vi "joystick+serial to robot.vi"() -> ()   [LabVIEW 2016]
uses:
  grSim/grSim Robot Command.ctl
  <vilib>/Instr/_visa.llb/VISA Configure Serial Port (Instr).vi
panel:
  out "output cluster":T1
  out "return count":u32
  in  "stop":bool
  out "string":string
  out "error out":errorcluster
  in  "termination char\n(0xA = '\\n' = LF)":u8=10 format="%.0x"
  in  "VISA resource name":refnum<visa-resource-name>
  in  "Serial Settings":T2={"baud rate"=9600, "data bits"=8, "parity"=enum."None", "stop bits"=10, "flow control"=0} {"flow control" items=["None"=0, "XON/XOFF"=1, "RTS/CTS"=2, "DTR/DSR"=4]; "stop bits" items=["1.0"=10, "1.5"=15, "2.0"=20]; "data bits" min=5 max=8 step=1; "baud rate" items=["75"=75, "110"=110, "134"=134, "150"=150, "300"=300, "600"=600, "1200"=1200, "1800"=1800, "2400"=2400, "4800"=4800, "7200"=7200, "9600"=9600, "14400"=14400, "19200"=19200, "28800"=28800, "38400"=38400, "56000"=56000, "57600"=57600, "115200"=115200, "128000"=128000, "230400"=230400]}
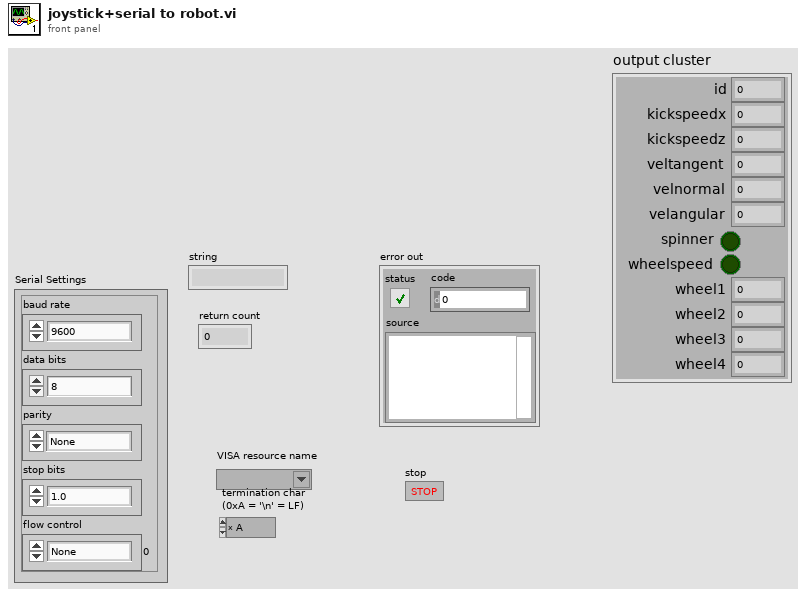
[diagram p1: front panel]
types:
  T1 = typedef "grSim Robot Command.ctl" = cluster{"id":u32, "kickspeedx":sgl, "kickspeedz":sgl, "veltangent":sgl, "velnormal":sgl, "velangular":sgl, "spinner":bool, "wheelspeed":bool, "wheel1":sgl, "wheel2":sgl, "wheel3":sgl, "wheel4":sgl}
  T2 = cluster{"baud rate":u32, "data bits":u16, "parity":enum16{"None", "Odd", "Even", "Mark", "Space"}, "stop bits":u16, "flow control":u16}
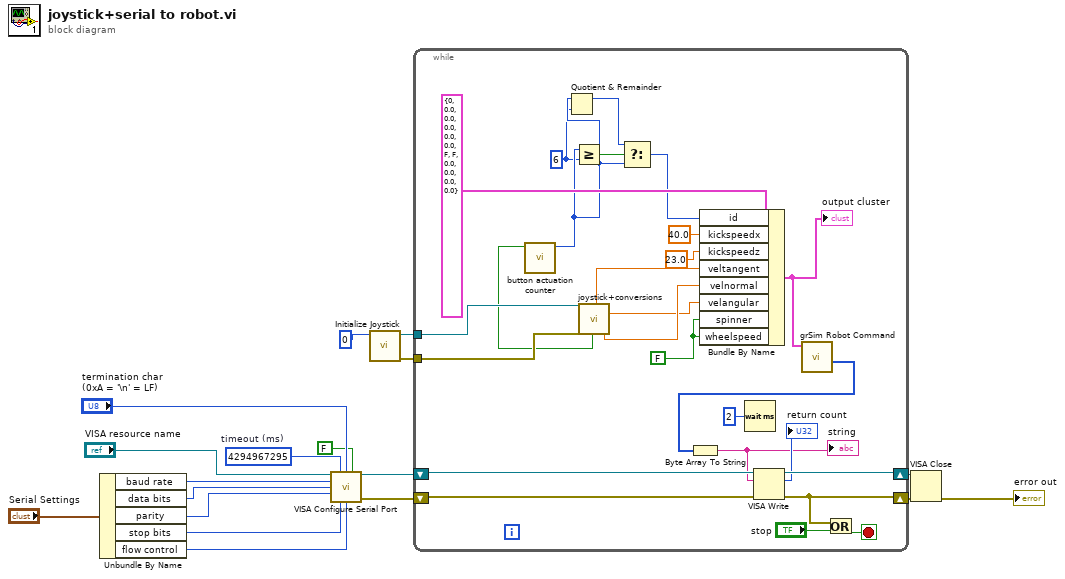
[diagram p0: block diagram]
diagram:
  w4 = u32 4294967295  # timeout (ms)
  n1 = Unbundle By Name("Serial Settings") -> ("baud rate"=w17:u32, "data bits"=w16:u16, "parity"=w15:enum16{"None", "Odd", "Even", "Mark", "Space"}, "stop bits"=w14:u16, "flow control"=w13:u16)
  n2 = call-poly "VISA Configure Serial Port"("VISA resource name"="VISA resource name", "timeout (10sec)"=w4, "termination char\n(0xA = '\\n' = LF)"="termination char\n(0xA = '\\n' = LF)", "Enable Termination\nChar (T)"=FALSE ("Enable Termination\nChar (T)"), "baud rate (9600)"=w17, "data bits (8)"=w16, "parity (0:none)"=w15, "stop bits (10: 1 bit)"=w14, "flow control (0:none)"=w13) -> ("VISA resource name out"=w9:refnum<visa-resource-name>, "error out"=w7:errorcluster)  [unwired: 5 in]
  n3 = call <vilib>:"Initialize Joystick.vi"("device index"=0) -> ("error out"=w1:errorcluster, "device ID"=w2:refnum<k1>)  [unwired: 9 in]
  n4 = while {
    shift-right: [w43] -> w8
    shift-left: w9 -> [w44]
    shift-right: [w38] -> w6
    shift-left: w7 -> [w42]
    tunnel: w2 -> [w27]
    tunnel: w1 -> [w26]
    stop <- w39 stop-if-true
    w20 = 6 ("y")
    w28 = FALSE
    n5 = call "joystick+conversions.vi"("Refnum in"=w27, "error in (no error)"=w26) -> ("B pressed"=w24:bool, "v_radial"=w29:dbl, "v_normal"=w31:dbl, "R*w"=w30:dbl)  [unwired: 9 in, 13 out]
    n6 = call "button actuation counter.vi"("button pressed"=w24) -> ("counter"=w21:i32)  [unwired: 10 in]
    n7 = Quotient & Remainder(x=w21, y=w20) -> (x-y*floor(x/y)=w19:i32)  [unwired: 1 out]
    n8 = Greater Or Equal?(x=w21, y=w20) -> (x >= y?=w23:bool)
    n9 = Select(t=w19, s=w23, f=w21) -> (s? t:f=w22:i32)
    n10 = Bundle By Name(cluster=T1 {"id"=0, "kickspeedx"=0.0, "kickspeedz"=0.0, "veltangent"=0.0, "velnormal"=0.0, "velangular"=0.0, "spinner"=FALSE, "wheelspeed"=FALSE, "wheel1"=0.0, "wheel2"=0.0, "wheel3"=0.0, "wheel4"=0.0} ("Robots"), "id"=w22, "kickspeedx"=sgl 40.0, "kickspeedz"=sgl 23.0 ("kickspeedx"), "veltangent"=w29, "velnormal"=w31, "velangular"=w30, "spinner"=w28, "wheelspeed"=w28) -> (w25:T1)
    "output cluster" <- w25
    n11 = Wait (ms)(milliseconds to wait=u32 2) -> ()  [unwired: 1 out]
    n12 = call "grSim Robot Command.vi"("Robots"=w25) -> ("Array"=w35:u8[])  [unwired: 10 in]
    n13 = Byte Array To String(unsigned byte array=w35) -> (string=w36:string)
    "string" <- w36
    n14 = VISA Write(VISA resource name=w44, write buffer=w36, error in (no error)=w42) -> (VISA resource name out=w43:refnum<visa-resource-name>, return count=→"return count":u32, error out=w38:errorcluster)
    n15 = Or(x=w38, y="stop") -> (x .or. y?=w39:bool)
  }
  n16 = VISA Close(VISA resource name=w8, error in (no error)=w6) -> (error out=→"error out":errorcluster)
